vi "TestDecoding.vi"() -> ()   [LabVIEW 2019]
uses:
  TypeDefs/TimeSymbol.ctl
panel:
  out "WWVB":u64 format="%.0x"
  out "Numeric":i32
  # "10C2708D0210823"
  # "1182708D0210825"
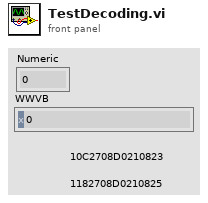
[diagram p1: front panel]
types:
  T1 = typedef "TimeSymbol.ctl" = enum16{"0", "1", "Marker", "Invalid"}
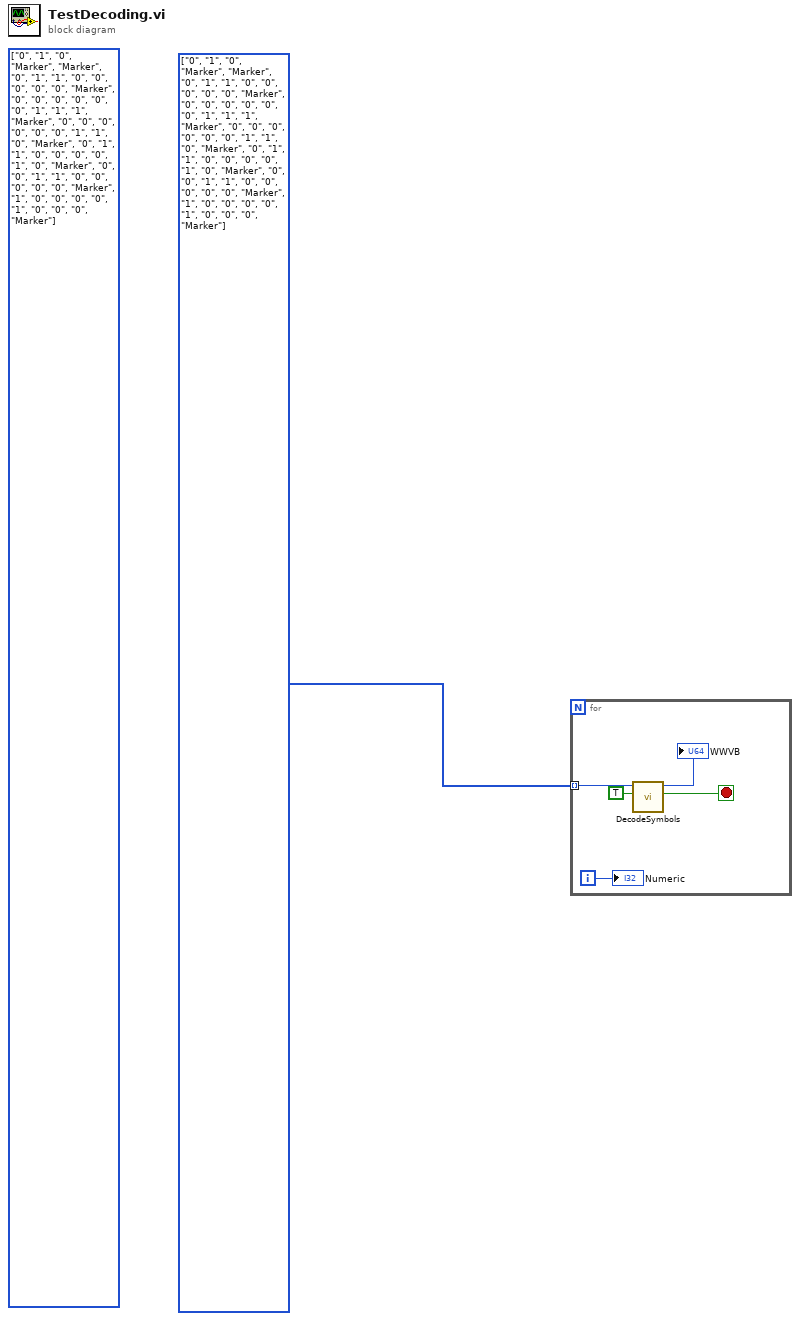
[diagram p0: block diagram]
diagram:
  (unwired) T1[] [enum."0", enum."1", enum."0", enum."Marker", enum."Marker", enum."0", enum."1", enum."1", enum."0", enum."0", enum."0", enum."0", enum."0", enum."Marker", enum."0", enum."0", enum."0", enum."0", enum."0", enum."0", enum."1", enum."1", enum."1", enum."Marker", enum."0", enum."0", enum."0", enum."0", enum."0", enum."0", enum."1", enum."1", enum."0", enum."Marker", enum."0", enum."1", enum."1", enum."0", enum."0", enum."0", enum."0", enum."1", enum."0", enum."Marker", enum."0", enum."0", enum."1", enum."1", enum."0", enum."0", enum."0", enum."0", enum."0", enum."Marker", enum."1", enum."0", enum."0", enum."0", enum."0", enum."1", enum."0", enum."0", enum."0", enum."Marker"] items=["0", "1", "Marker", "Invalid"]
  w1 = T1[] [enum."0", enum."1", enum."0", enum."Marker", enum."Marker", enum."0", enum."1", enum."1", enum."0", enum."0", enum."0", enum."0", enum."0", enum."Marker", enum."0", enum."0", enum."0", enum."0", enum."0", enum."0", enum."1", enum."1", enum."1", enum."Marker", enum."0", enum."0", enum."0", enum."0", enum."0", enum."0", enum."1", enum."1", enum."0", enum."Marker", enum."0", enum."1", enum."1", enum."0", enum."0", enum."0", enum."0", enum."1", enum."0", enum."Marker", enum."0", enum."0", enum."1", enum."1", enum."0", enum."0", enum."0", enum."0", enum."0", enum."Marker", enum."1", enum."0", enum."0", enum."0", enum."0", enum."1", enum."0", enum."0", enum."0", enum."Marker"] items=["0", "1", "Marker", "Invalid"]
  n1 = for {
    tunnel: w1 -> [w6] mode=indexing
    i -> [w4]
    stop <- w3 stop-if-true
    n2 = call "DecodeSymbols.vi"("InputValid"=TRUE, "Symbol"=w6) -> ("Output Valid"=w3:bool, "WWVB"=→"WWVB":u64)  [unwired: 8 in]
    "Numeric" <- w4
  }
